vi "Power Settings.vi"(8 "error in (no error)":errorcluster, 10 "File Path Control":path, 11 "Power Analyzer":T1=enum."APLUS") -> (0 "error out":errorcluster, 2 "Power Analyzer Out":T1=enum."APLUS", 3 "Power Out":T2={"Yokogawa"={"WT210"={"Sample Rate (1: 0.25s)"=1, "A Range (12: 20A)"=11, "V Range (6: 600V)"=4, "Power VISA Yokogawa WT210"=""}, "WT500"={"Power VISA Yokogawa WT500"="", "V Range (8: 1000V)"=6, "I Range (7: 40A)"=7, "Update Rate (3: 500ms)"=2}}, "Aplus"={"Aplus IP Address"="192.168.1.101", "Remote Port"=502, "Instrument"="APLUS", "Instr Driver Revision"="1.03.0053"}, "Power Limits"={"Crest Factor"={"Upper Limit"=1.49, "Lower Limit"=1.34}, "Harmonic Content"={"Uthd"=2.0}, "Voltage"={"% Error"=2.0}, "Stability"={"<1 Watt "={"Wattage"=1.0, "Slope (mW/H)"=10.0}, ">1 Watt"={"1%Power/Hour"=1.0}}}, "Nominal Voltage"=120, "Time Limit (s)"=10800.0, "Power Variation Limit (%)"=50.0, "Power Supply"={"Chroma 61605"="CHROMA", "Use Chroma?"=FALSE}} {"Yokogawa"."WT500"."Update Rate (3: 500ms)" items=["-", "100ms", "200ms", "500ms", "1s", "2s", "5s"]; "Yokogawa"."WT500"."I Range (7: 40A)" items=["AUTO", "500 mA", "1 A", "2 A", "5 A", "10 A", "20 A", "40 A", "S-AUTO", "50 mV", "100 mV", "200 mV", "500 mV", "1 V", "2 V", "5 V", "10 V", "250 mA", "500 mA", "1 A", "2.5 A", "5 A", "10 A", "20 A", "25 mV", "50 mV", "100 mV", "250 mV", "500 mV", "1 V", "2.5 V", "5 V"]; "Yokogawa"."WT500"."V Range (8: 1000V)" items=["AUTO", "15", "30", "60", "100", "150", "300", "600", "1000", "7.5", "15", "30", "50", "75", "150", "300", "500"]; "Yokogawa"."WT210"."V Range (6: 600V)" items=["Auto", "15V", "30V", "60V", "150V", "300V", "600V"]; "Yokogawa"."WT210"."A Range (12: 20A)" items=["Auto", "5mA", "10mA", "20mA", "50mA", "100mA", "200mA", "0.5A", "1A", "2A", "5A", "10A", "20A", "50mV", "100mV", "200mV", "2.5V", "5V", "10V"]; "Yokogawa"."WT210"."Sample Rate (1: 0.25s)" items=["0.1s", "0.25s", "0.5s", "1s", "2s", "5s"]})   [LabVIEW 2016]
uses:
  Type Definitions/UTILITY Power Inputs Control.ctl
  Type Definitions/UTILITY Power Analyzer.ctl
  <vilib>/Instr/_visa.llb/VISA Find Search Mode.ctl
  <vilib>/Utility/file.llb/Read From Spreadsheet File (string).vi
panel:
  in  "Update Rate (3: 500ms)":u16(ring)=2 items=["-", "100ms", "200ms", "500ms", "1s", "2s", "5s"]
  in  "I Range (7: 40A)":u16(ring)=7 items=["AUTO", "500 mA", "1 A", "2 A", "5 A", "10 A", "20 A", "40 A", "S-AUTO", "50 mV", "100 mV", "200 mV", "500 mV", "1 V", "2 V", "5 V", "10 V", "250 mA", "500 mA", "1 A", "2.5 A", "5 A", "10 A", "20 A", "25 mV", "50 mV", "100 mV", "250 mV", "500 mV", "1 V", "2.5 V", "5 V"]
  in  "V Range (8: 1000V)":u16(ring)=6 items=["AUTO", "15", "30", "60", "100", "150", "300", "600", "1000", "7.5", "15", "30", "50", "75", "150", "300", "500"]
  in  "Sample Rate (1: 0.25s)":i32(ring)=1 items=["0.1s", "0.25s", "0.5s", "1s", "2s", "5s"]
  in  "A Range (12: 20A)":i32(ring)=11 items=["Auto", "5mA", "10mA", "20mA", "50mA", "100mA", "200mA", "0.5A", "1A", "2A", "5A", "10A", "20A", "50mV", "100mV", "200mV", "2.5V", "5V", "10V"]
  in  "V Range (6: 600V)":i32(ring)=4 items=["Auto", "15V", "30V", "60V", "150V", "300V", "600V"]
  in  "Power IN":T2={"Yokogawa"={"WT210"={"Sample Rate (1: 0.25s)"=1, "A Range (12: 20A)"=11, "V Range (6: 600V)"=4, "Power VISA Yokogawa WT210"=""}, "WT500"={"Power VISA Yokogawa WT500"="", "V Range (8: 1000V)"=6, "I Range (7: 40A)"=7, "Update Rate (3: 500ms)"=2}}, "Aplus"={"Aplus IP Address"="192.168.1.101", "Remote Port"=502, "Instrument"="APLUS", "Instr Driver Revision"="1.03.0053"}, "Power Limits"={"Crest Factor"={"Upper Limit"=1.49, "Lower Limit"=1.34}, "Harmonic Content"={"Uthd"=2.0}, "Voltage"={"% Error"=2.0}, "Stability"={"<1 Watt "={"Wattage"=1.0, "Slope (mW/H)"=10.0}, ">1 Watt"={"1%Power/Hour"=1.0}}}, "Nominal Voltage"=120, "Time Limit (s)"=10800.0, "Power Variation Limit (%)"=50.0, "Power Supply"={"Chroma 61605"="CHROMA", "Use Chroma?"=FALSE}} {"Yokogawa"."WT500"."Update Rate (3: 500ms)" items=["-", "100ms", "200ms", "500ms", "1s", "2s", "5s"]; "Yokogawa"."WT500"."I Range (7: 40A)" items=["AUTO", "500 mA", "1 A", "2 A", "5 A", "10 A", "20 A", "40 A", "S-AUTO", "50 mV", "100 mV", "200 mV", "500 mV", "1 V", "2 V", "5 V", "10 V", "250 mA", "500 mA", "1 A", "2.5 A", "5 A", "10 A", "20 A", "25 mV", "50 mV", "100 mV", "250 mV", "500 mV", "1 V", "2.5 V", "5 V"]; "Yokogawa"."WT500"."V Range (8: 1000V)" items=["AUTO", "15", "30", "60", "100", "150", "300", "600", "1000", "7.5", "15", "30", "50", "75", "150", "300", "500"]; "Yokogawa"."WT210"."V Range (6: 600V)" items=["Auto", "15V", "30V", "60V", "150V", "300V", "600V"]; "Yokogawa"."WT210"."A Range (12: 20A)" items=["Auto", "5mA", "10mA", "20mA", "50mA", "100mA", "200mA", "0.5A", "1A", "2A", "5A", "10A", "20A", "50mV", "100mV", "200mV", "2.5V", "5V", "10V"]; "Yokogawa"."WT210"."Sample Rate (1: 0.25s)" items=["0.1s", "0.25s", "0.5s", "1s", "2s", "5s"]}
  out "all rows":string[][](array[string])
  # "WT210"
  # "WT500"
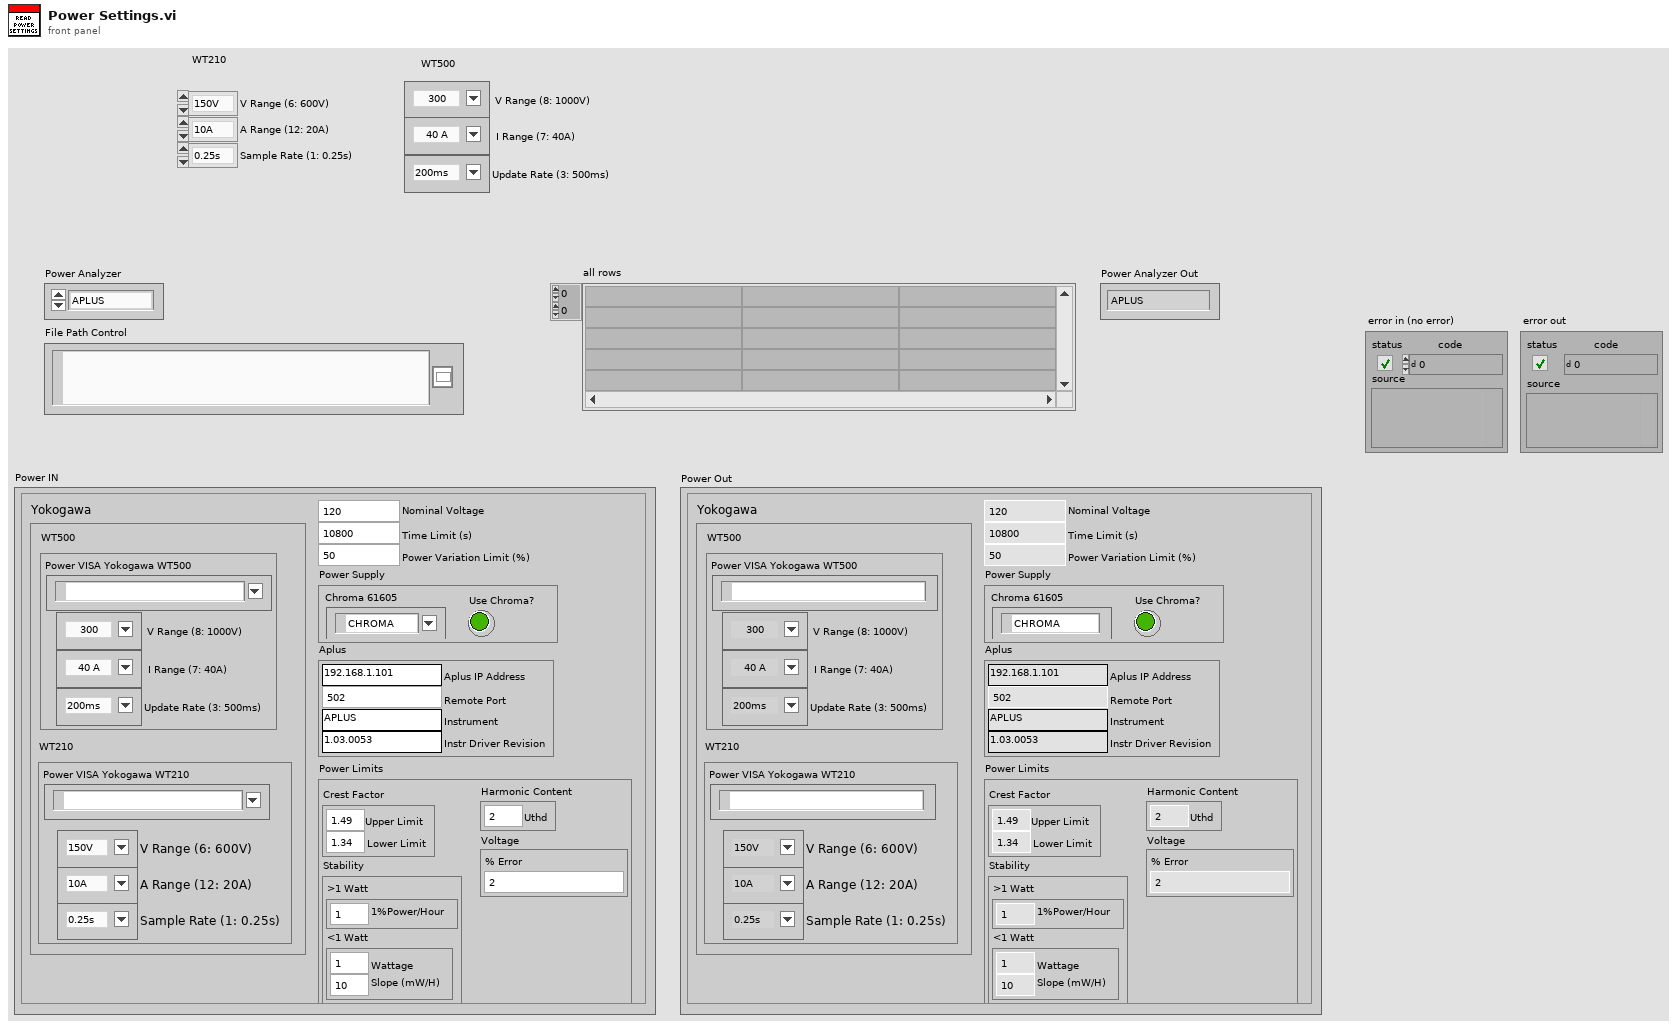
[diagram p1: front panel]
types:
  T1 = typedef "UTILITY Power Analyzer.ctl" = enum16{"", "APLUS", "WT210", "WT500", "WT300", "OSI", "Debug", "WT230"}
  T2 = typedef "UTILITY Power Inputs Control.ctl" = cluster{"Yokogawa":cluster{"WT210":cluster{"Sample Rate (1: 0.25s)":i32, "A Range (12: 20A)":i32, "V Range (6: 600V)":i32, "Power VISA Yokogawa WT210":refnum<visa-resource-name>}, "WT500":cluster{"Power VISA Yokogawa WT500":refnum<visa-resource-name>, "V Range (8: 1000V)":i32, "I Range (7: 40A)":i32, "Update Rate (3: 500ms)":i32}}, "Aplus":cluster{"Aplus IP Address":string, "Remote Port":i32, "Instrument":string, "Instr Driver Revision":string}, "Power Limits":cluster{"Crest Factor":cluster{"Upper Limit":dbl, "Lower Limit":dbl}, "Harmonic Content":cluster{"Uthd":dbl}, "Voltage":cluster{"% Error":dbl}, "Stability":cluster{"<1 Watt ":cluster{"Wattage":dbl, "Slope (mW/H)":dbl}, ">1 Watt":cluster{"1%Power/Hour":dbl}}}, "Nominal Voltage":i32, "Time Limit (s)":dbl, "Power Variation Limit (%)":dbl, "Power Supply":cluster{"Chroma 61605":refnum<visa-resource-name>, "Use Chroma?":bool}}
  T3 = typedef "VISA Find Search Mode.ctl" = u32
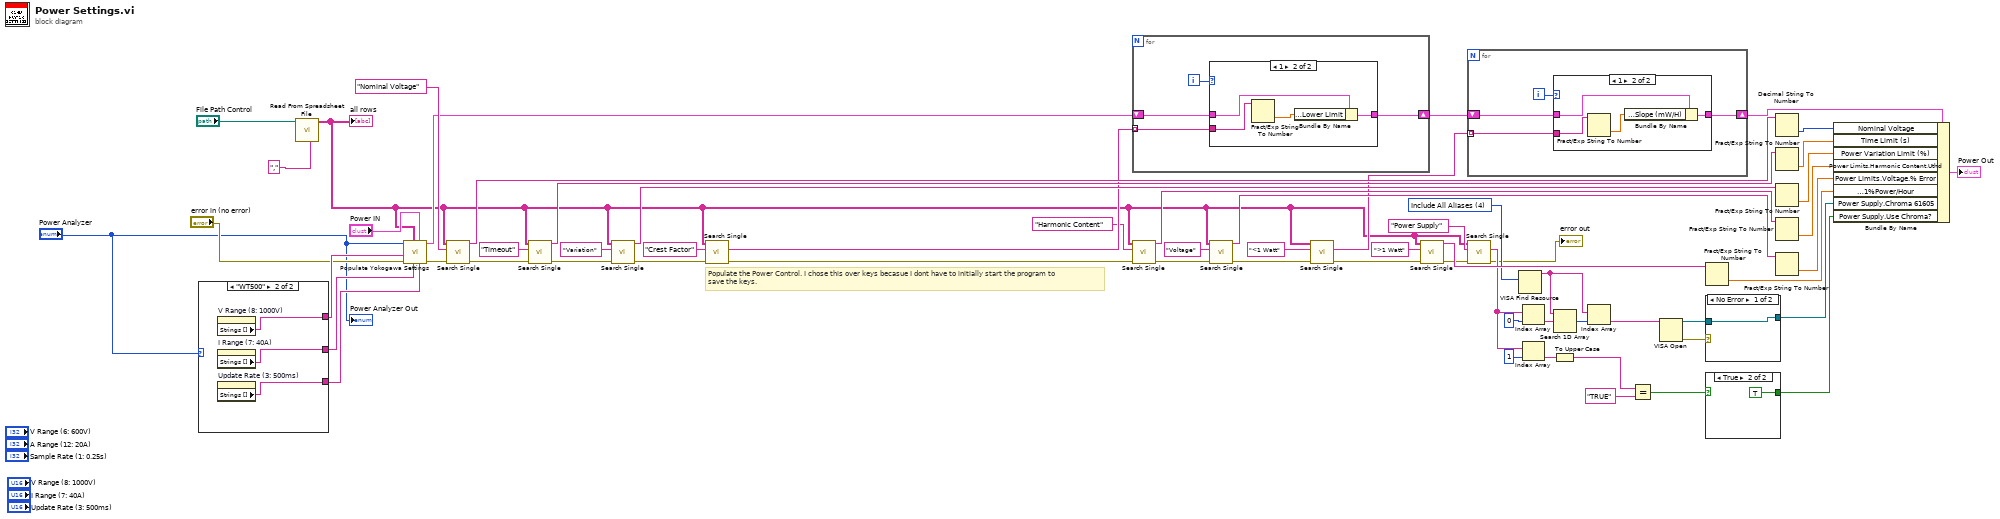
[diagram p0: block diagram]
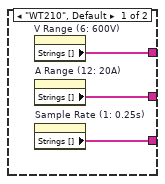
[diagram p2: hidden frame]
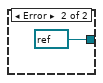
[diagram p3: hidden frame]
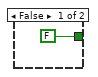
[diagram p4: hidden frame]
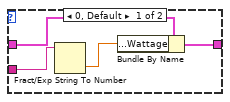
[diagram p5: hidden frame]
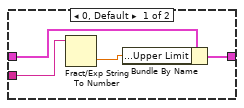
[diagram p6: hidden frame]
diagram:
  w19 = T3 4 items=["Canonical Names Only"=0, "Aliases Only"=2, "Include Matching Aliases"=3, "Include All Aliases"=4] ("Search Mode")
  # "Populate the Power Control. I chose this over keys becasue I dont have to initially start the program to\nsave the keys."
  n1 = case shown="\"WT500\"" "Power Analyzer" {
    tunnel: [w65 w68] -> w59
    tunnel: [w64 w67] -> w58
    tunnel: [w63 w66] -> w57
    frame "WT210", Default {
      n2 = property on="V Range (6: 600V)" class="Ring (strict)"() -> ("Strings []"=w65:string[])  [unwired: 2 in, 2 out]
      n3 = property on="A Range (12: 20A)" class="Ring (strict)"() -> ("Strings []"=w64:string[])  [unwired: 2 in, 2 out]
      n4 = property on="Sample Rate (1: 0.25s)" class="Ring (strict)"() -> ("Strings []"=w63:string[])  [unwired: 2 in, 2 out]
    }
    frame "WT500" {
      n5 = property on="V Range (8: 1000V)" class="Ring (strict)"() -> ("Strings []"=w68:string[])  [unwired: 2 in, 2 out]
      n6 = property on="I Range (7: 40A)" class="Ring (strict)"() -> ("Strings []"=w67:string[])  [unwired: 2 in, 2 out]
      n7 = property on="Update Rate (3: 500ms)" class="Ring (strict)"() -> ("Strings []"=w66:string[])  [unwired: 2 in, 2 out]
    }
  }
  n8 = call-poly <vilib>:"Read From Spreadsheet File.vi"("delimiter (\\t)"="," ("delimiter (\\t)"), "file path (dialog if empty)"="File Path Control") -> ("all rows"=w16:string[][])  [unwired: 5 in, 4 out]
  "all rows" <- w16
  n9 = call "Populate Yokogawa Settings.vi"("Sample Rate"=w57, "Power  in"="Power IN", "A Range"=w58, "Input Array"=w16, "error in (no error)"="error in (no error)", "V Range"=w59, "Power Analyzer"="Power Analyzer") -> ("error out"=w53:errorcluster, "Power  out"=w41:T2)  [unwired: 3 in]
  n10 = call "Search Single.vi"("error in (no error)"=w53, "Search"="Nominal Voltage" ("delimiter (\\t)"), "all rows"=w16) -> ("error out"=w52:errorcluster, "Output"=w50:string)  [unwired: 6 in, 1 out]
  n11 = call "Search Single.vi"("error in (no error)"=w52, "Search"="Timeout" ("delimiter (\\t)"), "all rows"=w16) -> ("error out"=w51:errorcluster, "Output"=w48:string)  [unwired: 6 in, 1 out]
  n12 = call "Search Single.vi"("error in (no error)"=w51, "Search"="Variation" ("delimiter (\\t)"), "all rows"=w16) -> ("error out"=w40:errorcluster, "Output"=w46:string)  [unwired: 6 in, 1 out]
  n13 = call "Search Single.vi"("error in (no error)"=w40, "Search"="Crest Factor", "all rows"=w16) -> ("error out"=w33:errorcluster, "Array Output"=w42:string[])  [unwired: 6 in, 1 out]
  n14 = for {
    tunnel: w42 -> [w72] mode=indexing
    shift-right: [w69] -> w29
    shift-left: w41 -> [w70]
    i -> [w71]
    n15 = case shown="1" w71 {
      tunnel: w72 -> [w74 w78]
      tunnel: w70 -> [w76 w80]
      tunnel: [w75 w79] -> w69
      frame 0, Default {
        n16 = Fract/Exp String To Number(string=w74) -> (number=w73:dbl)  [unwired: 3 in, 1 out]
        n17 = Bundle By Name(cluster=w76, "Power Limits.Crest Factor.Upper Limit"=w73) -> (w75:T2)
      }
      frame 1 {
        n18 = Fract/Exp String To Number(string=w78) -> (number=w77:dbl)  [unwired: 3 in, 1 out]
        n19 = Bundle By Name(cluster=w80, "Power Limits.Crest Factor.Lower Limit"=w77) -> (w79:T2)
      }
    }
  }
  n20 = call "Search Single.vi"("error in (no error)"=w33, "Search"="Harmonic Content", "all rows"=w16) -> ("error out"=w32:errorcluster, "Output"=w37:string)  [unwired: 6 in, 1 out]
  n21 = call "Search Single.vi"("error in (no error)"=w32, "Search"="Voltage", "all rows"=w16) -> ("error out"=w24:errorcluster, "Output"=w36:string)  [unwired: 6 in, 1 out]
  n22 = call "Search Single.vi"("error in (no error)"=w24, "Search"="<1 Watt", "all rows"=w16) -> ("error out"=w23:errorcluster, "Array Output"=w28:string[])  [unwired: 6 in, 1 out]
  n23 = call "Search Single.vi"("error in (no error)"=w23, "Search"=">1 Watt", "all rows"=w16) -> ("error out"=w18:errorcluster, "Output"=w26:string)  [unwired: 6 in, 1 out]
  n24 = for {
    tunnel: w28 -> [w84] mode=indexing
    shift-right: [w81] -> w27
    shift-left: w29 -> [w82]
    i -> [w83]
    n25 = case shown="1" w83 {
      tunnel: w84 -> [w86 w90]
      tunnel: w82 -> [w88 w92]
      tunnel: [w87 w91] -> w81
      frame 0, Default {
        n26 = Fract/Exp String To Number(string=w86) -> (number=w85:dbl)  [unwired: 3 in, 1 out]
        n27 = Bundle By Name(cluster=w88, "Power Limits.Stability.<1 Watt.Wattage"=w85) -> (w87:T2)
      }
      frame 1 {
        n28 = Fract/Exp String To Number(string=w90) -> (number=w89:dbl)  [unwired: 3 in, 1 out]
        n29 = Bundle By Name(cluster=w92, "Power Limits.Stability.<1 Watt.Slope (mW/H)"=w89) -> (w91:T2)
      }
    }
  }
  n30 = call "Search Single.vi"("error in (no error)"=w18, "Search"="Power Supply", "all rows"=w16) -> ("error out"=→"error out":errorcluster, "Array Output"=w12:string[])  [unwired: 6 in, 1 out]
  n31 = VISA Find Resource(10:w19) -> (3:w21:string[])  [unwired: 2 in, 2 out]
  n32 = Index Array(array=w12, index=0) -> (element=w14:string)
  n33 = Index Array(array=w12, index=1) -> (element=w8:string)
  n34 = To Upper Case(1:w8) -> (0:w9:string)
  n35 = Search 1D Array(1D array=w21, element=w14) -> (index of element=w20:i32)  [unwired: 1 in]
  n36 = Index Array(array=w21, index=w20) -> (element=w22:string)
  n37 = Equal?(x=w9, y="TRUE") -> (x = y?=w11:bool)
  n38 = VISA Open(VISA resource name=w22) -> (VISA resource name=w6:refnum<visa-resource-name>, error out=w4:errorcluster)  [unwired: 4 in]
  n39 = Fract/Exp String To Number(string=w26) -> (number=w25:dbl)  [unwired: 3 in, 1 out]
  n40 = case shown="No Error" w4 {
    tunnel: [w93 refnum<visa-resource-name> refnum ("VISA resource name")] -> w5
    tunnel: w6 -> [w93 _]
    frame No Error {
    }
    frame Error {
    }
  }
  n41 = case shown="True" w11 {
    tunnel: [FALSE TRUE] -> w7
    frame False {
    }
    frame True {
    }
  }
  n42 = Decimal String To Number(string=w50) -> (number=w49:i32)  [unwired: 2 in, 1 out]
  n43 = Fract/Exp String To Number(string=w48) -> (number=w47:dbl)  [unwired: 3 in, 1 out]
  n44 = Fract/Exp String To Number(string=w46) -> (number=w45:dbl)  [unwired: 3 in, 1 out]
  n45 = Fract/Exp String To Number(string=w37) -> (number=w35:dbl)  [unwired: 3 in, 1 out]
  n46 = Fract/Exp String To Number(string=w36) -> (number=w34:dbl)  [unwired: 3 in, 1 out]
  n47 = Bundle By Name(cluster=w27, "Nominal Voltage"=w49, "Time Limit (s)"=w47, "Power Variation Limit (%)"=w45, "Power Limits.Harmonic Content.Uthd"=w35, "Power Limits.Voltage.% Error"=w34, "Power Limits.Stability.>1 Watt.1%Power/Hour"=w25, "Power Supply.Chroma 61605"=w5, "Power Supply.Use Chroma?"=w7) -> (→"Power Out":T2)
  "Power Analyzer Out" <- "Power Analyzer"
